vi "Create device from VISA.vi"(6 "Sub Panel":refnum<vi>, 8 "error in (no error)":errorcluster, 11 "VISA resource name":refnum<visa-resource-name>) -> (0 "error out":errorcluster, 2 "Device out":refnum<class "Instrument.lvclass">, 3 "VISA resource name out":refnum<visa-resource-name>)   [LabVIEW 2015]
uses:
  Instruments/Instrument/Instrument.lvclass
  Device/Device.lvclass
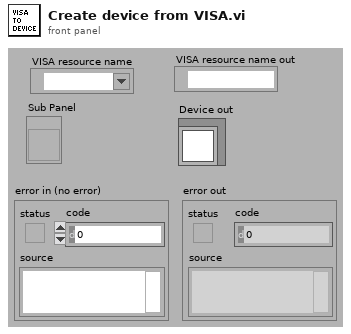
[diagram p1: front panel]
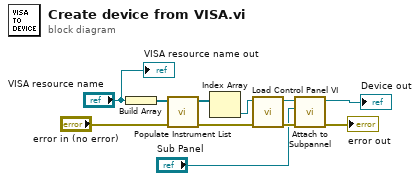
[diagram p0: block diagram]
diagram:
  n1 = Build Array("VISA resource name") -> (w10:refnum<visa-resource-name>[])
  n2 = call "Populate Instrument List.vi"("error in (no error)"="error in (no error)", "VISA Resourse Names"=w10) -> ("error out"=w5:errorcluster, "Instrument List"=w11:refnum<class "Instrument.lvclass">[])  [unwired: 2 in, 6 out]
  n3 = Index Array(array=w11) -> (element=w9:refnum<class "Instrument.lvclass">)  [unwired: 1 in]
  n4 = call "Load Control Panel VI.vi"("error in (no error)"=w5, "Device"=w9) -> ("error out"=w7:errorcluster, "Device out"=w8:refnum<class "Instrument.lvclass">)  [unwired: 7 in, 1 out]
  n5 = call "Attach to Subpannel.vi"("error in (no error)"=w7, "Sub Panel"="Sub Panel", "Device in"=w8) -> ("error out"=→"error out":errorcluster, "Device out"=→"Device out":refnum<class "Instrument.lvclass">)  [unwired: 7 in]
  "VISA resource name out" <- "VISA resource name"
